vi "Facade 1.vi"(0 "Data In":T5, 2 "Display State In":T3, 3 "Container State":T4) -> (6 "Data Out":T5, 7 "Display State Out":T3, 8 "Action":T2)   [LabVIEW 2011, in "Calculator XControl.xctl"]
doc: "This VI defines the appearance and behavior of the Calculator XControl. The front panel of the Facade VI defines the appearance of the XControl. The block diagram of the Facade VI describes the behavior of the XControl, using an Event Structure to define responses to various events that can occur on the XControl."
uses:
  Calculator XControl.xctl
  Data 1.ctl
  <vilib>/_xctls/Container State.ctl
  State 1.ctl
  <vilib>/_xctls/Action.ctl
  Controls/Format.ctl
  <vilib>/event_ctls.llb/eventvkey.ctl
  <vilib>/_xctls/XControlSupport.lvlib
  <vilib>/gmath/NI_Gmath.lvlib
panel:
  out "Output":string
  in  "Backspace":bool
  in  "(":bool
  in  ")":bool
  in  "^":bool
  in  "E":bool
  in  "Tab Control":enum32{"Func", "Symbol"}(tab)
  in  "Cot":bool
  in  "Csc":bool
  in  "Sec":bool
  in  "e^":bool
  in  "tanh":bool
  in  "cosh":bool
  in  "sinh":bool
  in  "log":bool
  in  "ln":bool
  in  "Tan":bool
  in  "Cos":bool
  in  "Sin":bool
  in  "NA":bool
  in  "R":bool
  in  "c":bool
  in  "exp":bool
  in  "pi":bool
  in  "Answer":bool
  in  "Clear":bool
  in  "Precision":u8=6
  in  "Format":T1 items=["Decimal"=0, "Scientific"=1, "Hexadecimal"=5]
  in  "Equals":bool
  in  "Nine":bool
  in  "Eight":bool
  in  "Seven":bool
  in  "Six":bool
  in  "Five":bool
  in  "Four":bool
  in  "Decimal":bool
  in  "Three":bool
  in  "Two":bool
  in  "Zero":bool
  in  "One":bool
  in  "Divide":bool
  in  "Multiply":bool
  in  "Minus":bool
  in  "Plus":bool
  in  "Formula":string
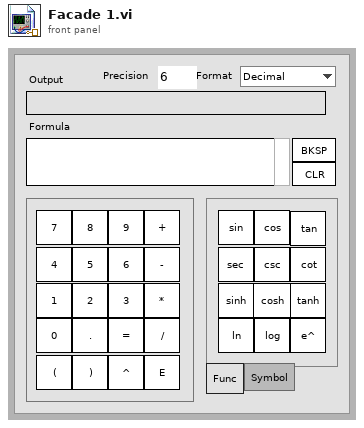
[diagram p1: front panel]
types:
  T1 = typedef "Calculator XControl.xctl/Format.ctl" = u16
  T2 = typedef "XControlSupport.lvlib/Action.ctl" = cluster{"Data Changed?":bool, "State Changed?":bool, "Action Name":string}
  T3 = typedef "Calculator XControl.xctl/State 1.ctl" = cluster{"Previous Formulas":string[]}
  T4 = typedef "XControlSupport.lvlib/Container State.ctl" = cluster{"Indicator?":bool, "Run Mode?":bool, " Refnum":refnum<vi>}
  T5 = typedef "Calculator XControl.xctl/Data 1.ctl" = dbl
  T6 = typedef "eventvkey.ctl" = enum16{"ASCII", "Enter", "Return", "Shift", "Ctrl", "Alt", "Cmd", "Opt", "Caps", "NumLock", "Clear", "Break", "Up", "Down", "Left", "Right", "Insert", "Delete", "Home", "End", "PageUp", "PageDown", "Escape", "Help", "Pause", "ScrollLock", "F1", "F2", "F3", "F4", "F5", "F6", "F7", "F8", "F9", "F10", "F11", "F12", "F13", "F14", "F15", "F16", "F17", "F18", "F19", "F20", "F21", "F22", "F23", "F24", "Play", "VolumeUp", "VolumeDown", "Mute", "Two Byte Char"}
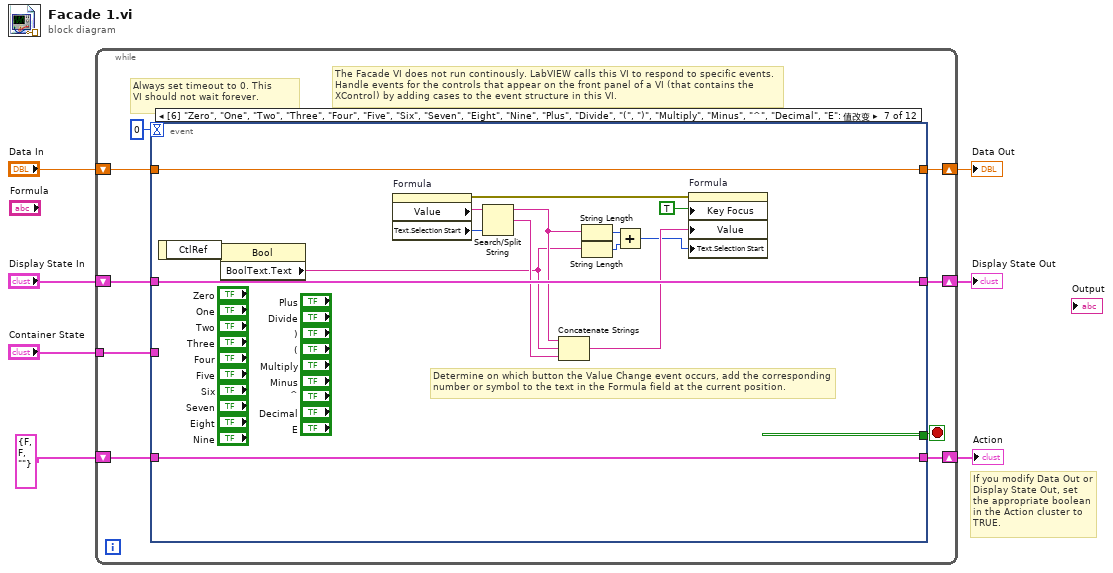
[diagram p0: block diagram]
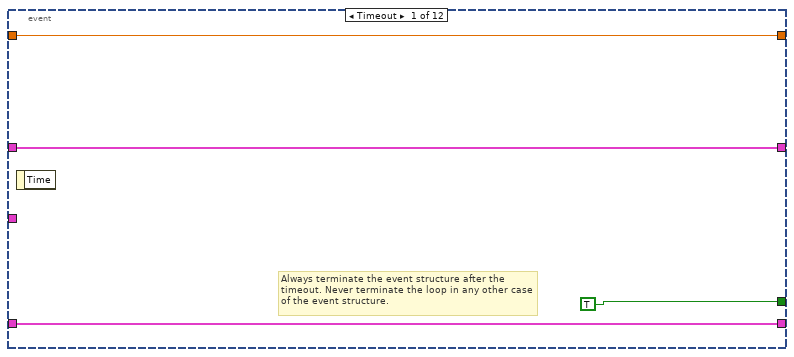
[diagram p2: hidden frame]
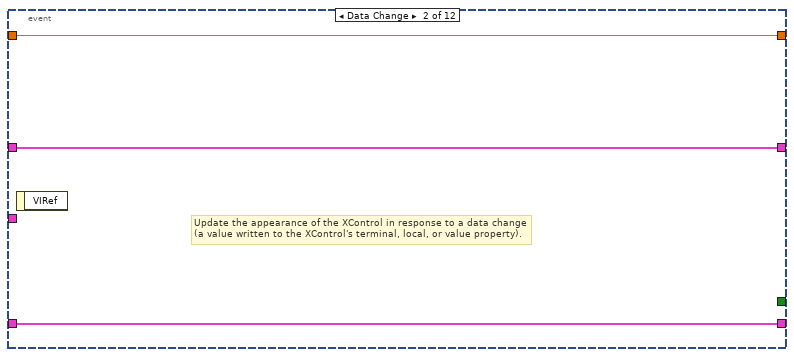
[diagram p3: hidden frame]
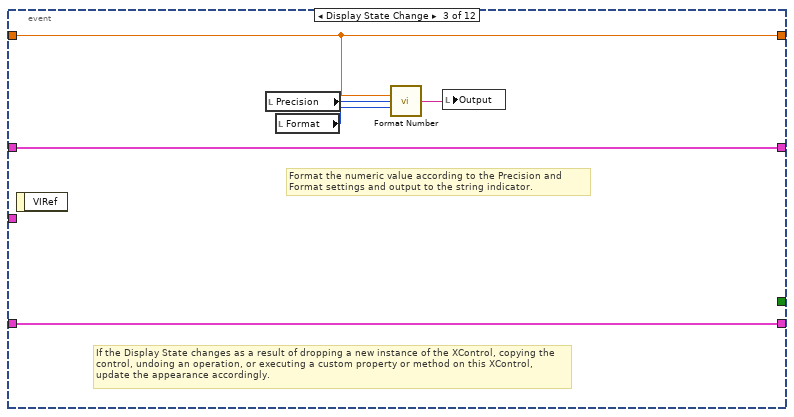
[diagram p4: hidden frame]
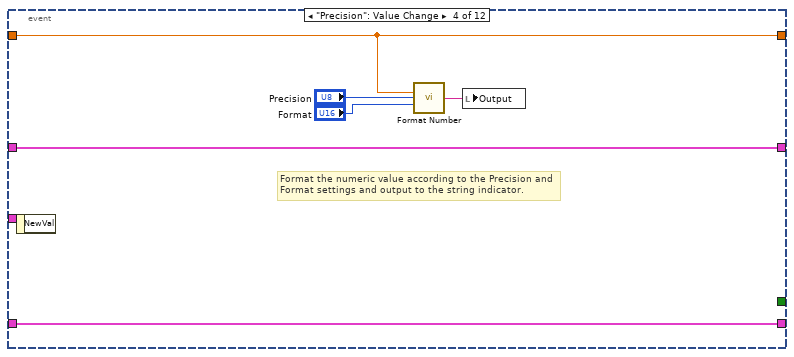
[diagram p5: hidden frame]
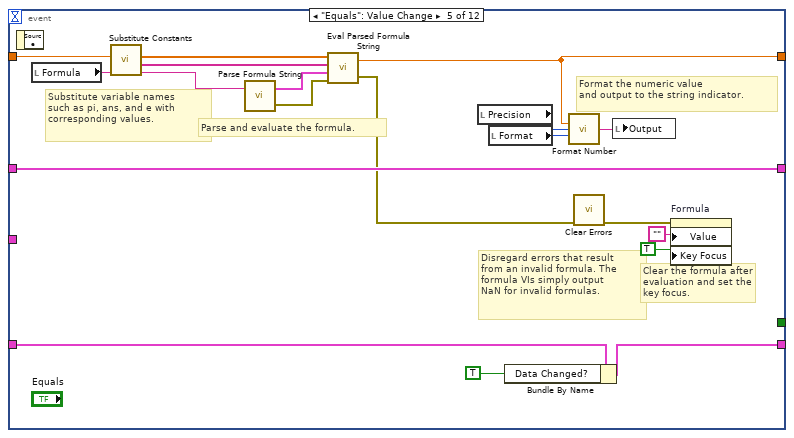
[diagram p6: hidden frame]
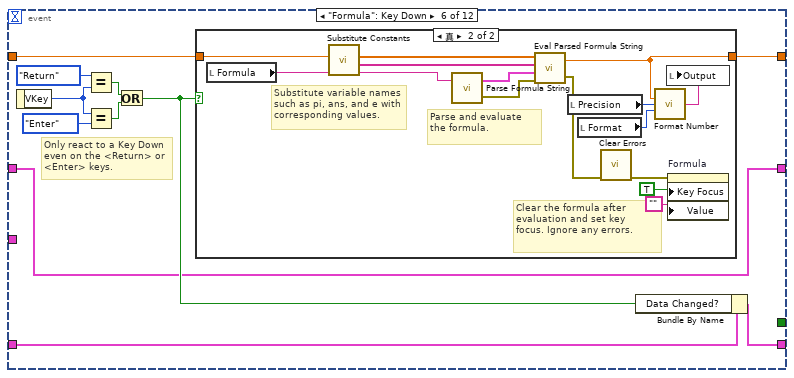
[diagram p7: hidden frame]
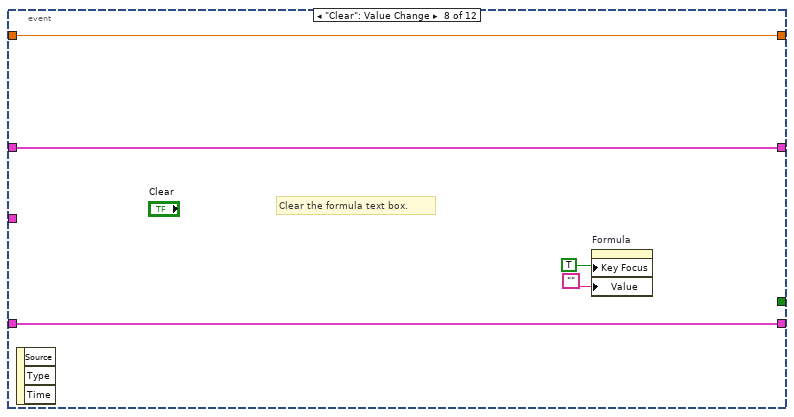
[diagram p9: hidden frame]
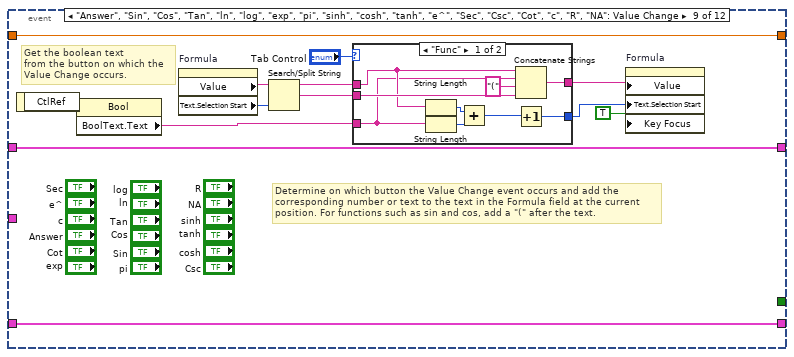
[diagram p10: hidden frame]
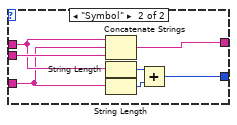
[diagram p11: hidden frame]
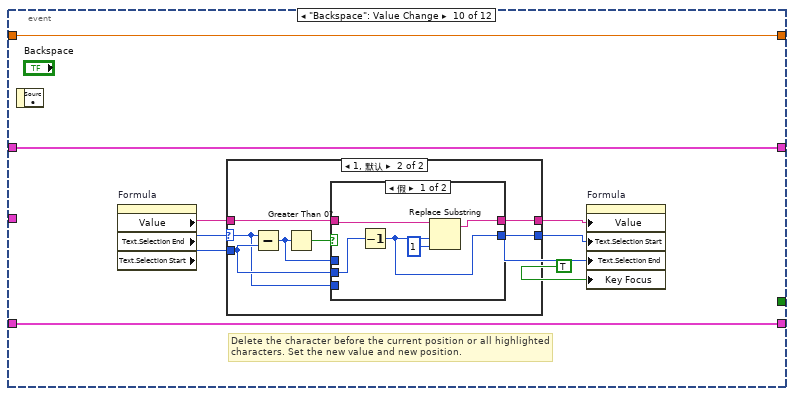
[diagram p12: hidden frame]
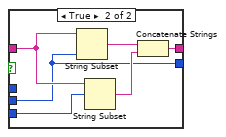
[diagram p14: hidden frame]
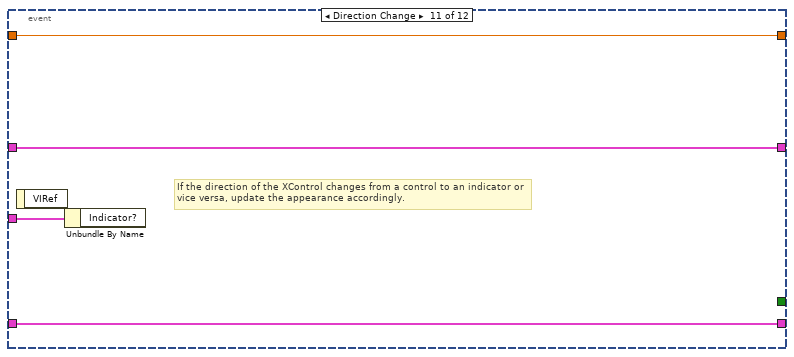
[diagram p15: hidden frame]
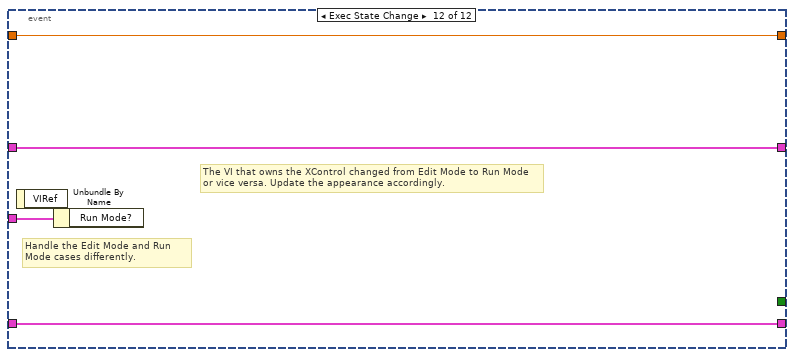
[diagram p16: hidden frame]
diagram:
  # "If you modify Data Out or Display State Out, set the appropriate boolean in the Action cluster to TRUE."
  n1 = while {
    shift-right: [w15] -> w4
    shift-left: "Display State In" -> [w16]
    tunnel: "Container State" -> [w12]
    shift-right: [w10] -> w7
    shift-left: "Data In" -> [w11]
    shift-right: [w8] -> w2
    shift-left: T2 {"Data Changed?"=FALSE, "State Changed?"=FALSE, "Action Name"=""} ("Action") -> [w9]
    stop <- w14 stop-if-true
    # "The Facade VI does not run continously. LabVIEW calls this VI to respond to specific events.  Handle events for the controls that appear on the front panel of a VI (that contains the XControl) by adding cases to the event structure in this VI."
    # "Always set timeout to 0. This\nVI should not wait forever."
    n2 = event shown="[6] \"Zero\", \"One\", \"Two\", \"Three\", \"Four\", \"Five\", \"Six\", \"Seven\", \"Eight\", \"Nine\", \"Plus\", \"Divide\", \"(\", \")\", \"Multiply\", \"Minus\", \"^\", \"Decimal\", \"E\": 值改变" {
      selector: _ -> [_ _ _ _ _ _ _ _ _ _ _ _]
      dyn-events: _ -> [_ _ _ _ _ _ _ _ _ _ _ _]
      timeout: 0 -> [_ _ _ _ _ _ _ _ _ _ _ _]
      tunnel: w16 -> [w18 w23 w28 w35 w42 w55 w95 w101 w113 w138 w162 w166]
      tunnel: [w18 w23 w28 w35 w42 w55 w95 w101 w113 w138 w162 w166] -> w15
      tunnel: [TRUE _ _ _ _ _ _ _ _ _ _ _] -> w14
      tunnel: w12 -> [_ _ _ _ _ _ _ _ _ _ w163 w167]
      tunnel: w11 -> [w17 w21 w27 w33 w47 w65 w94 w99 w114 w139 w161 w165]
      tunnel: [w17 w21 w27 w33 w37 w62 w94 w99 w114 w139 w161 w165] -> w10
      tunnel: [w19 w22 w29 w34 w51 w63 w96 w100 w112 w137 w160 w164] -> w8
      tunnel: w9 -> [w19 w22 w29 w34 w52 w64 w96 w100 w112 w137 w160 w164]
      event Timeout {
        # "Always terminate the event structure after the timeout. Never terminate the loop in any other case of the event structure."
        n3 = event-data() -> ()  [unwired: 1 in, 1 out]
      }
      event Data Change {
        # "Update the appearance of the XControl in response to a data change (a value written to the XControl's terminal, local, or value property)."
        n4 = event-data() -> ()  [unwired: 1 in, 1 out]
      }
      event Display State Change {
        # "Format the numeric value according to the Precision and Format settings and output to the string indicator."
        # "If the Display State changes as a result of dropping a new instance of the XControl, copying the control, undoing an operation, or executing a custom property or method on this XControl, update the appearance accordingly."
        n5 = event-data() -> ()  [unwired: 1 in, 1 out]
        n6 = local read "Precision"() -> (w25:u8)
        n7 = local read "Format"() -> (w26:T1)
        n8 = call "Format Number.vi"("Data"=w27, "precision (6)"=w25, "Format"=w26) -> ("Numeric String"=w24:string)  [unwired: 12 in]
        n9 = local write "Output"(w24) -> ()
      }
      event "Precision": Value Change {
        # "Format the numeric value according to the Precision and Format settings and output to the string indicator."
        n10 = event-data() -> ()  [unwired: 1 in, 1 out]
        n11 = call "Format Number.vi"("Data"=w33, "precision (6)"="Precision", "Format"="Format") -> ("Numeric String"=w30:string)  [unwired: 12 in]
        n12 = local write "Output"(w30) -> ()
      }
      event "Equals": Value Change {
        # "Format the numeric value\nand output to the string indicator."
        # "Disregard errors that result\nfrom an invalid formula. The\nformula VIs simply output\nNaN for invalid formulas."
        # "Clear the formula after\nevaluation and set the key focus."
        # "Parse and evaluate the formula."
        # "Substitute variable names\nsuch as pi, ans, and e with\ncorresponding values."
        n13 = event-data() -> ()  [unwired: 1 in, 1 out]
        n14 = local read "Formula"() -> (w44:string)
        n15 = call "Substitute Constants.vi"("Formula In"=w44, "Data In"=w47) -> ("Formula Out"=w43:string, "Variables Out"=w45:string[], "Values Out"=w46:dbl[])  [unwired: 7 in]
        n16 = call <vilib>:"Parse Formula String.vi"("formula"=w43) -> ("error out"=w54:errorcluster, "Parsed Formula"=w53:cluster{"Table":i32[][], "Y Values":dbl[]})  [unwired: 1 in]
        n17 = call <vilib>:"Eval Parsed Formula String.vi"("error in (no error)"=w54, "Parsed Formula"=w53, "Variables"=w45, "X Values"=w46) -> ("error out"=w41:errorcluster, "y value"=w37:dbl)
        n18 = local read "Precision"() -> (w38:u8)
        n19 = local read "Format"() -> (w39:T1)
        n20 = Bundle By Name(cluster=w52, "Data Changed?"=TRUE) -> (w51:T2)
        n21 = call "Format Number.vi"("Data"=w37, "precision (6)"=w38, "Format"=w39) -> ("Numeric String"=w36:string)  [unwired: 12 in]
        n22 = call <vilib>:"Clear Errors.vi"("error in (no error)"=w41) -> ("error out"=w40:errorcluster)  [unwired: 6 in]
        n23 = local write "Output"(w36) -> ()
        n24 = property on="Formula" class="Str"(error in=w40, "Value"="", "Key Focus"=TRUE) -> ()  [unwired: 1 in, 2 out]
      }
      event "Formula": Key Down {
        # "Only react to a Key Down even on the <Return> or <Enter> keys."
        n25 = event-data() -> ("VKey"=w60:T6)  [unwired: 1 in]
        n26 = Equal?(x=eventvkey."Return" ("y"), y=w60) -> (x = y?=w58:bool)
        n27 = Equal?(x=w60, y=eventvkey."Enter") -> (x = y?=w57:bool)
        n28 = Or(x=w58, y=w57) -> (x .or. y?=w56:bool)
        n29 = case shown="真" w56 {
          tunnel: w65 -> [w66 w77]
          tunnel: [w66 w70] -> w62
          frame False {
          }
          frame True {
            # "Clear the formula after\nevaluation and set key\nfocus. Ignore any errors."
            # "Substitute variable names\nsuch as pi, ans, and e with corresponding values."
            # "Parse and evaluate\nthe formula."
            n30 = local read "Formula"() -> (w74:string)
            n31 = call "Substitute Constants.vi"("Formula In"=w74, "Data In"=w77) -> ("Formula Out"=w73:string, "Variables Out"=w75:string[], "Values Out"=w76:dbl[])  [unwired: 7 in]
            n32 = call <vilib>:"Parse Formula String.vi"("formula"=w73) -> ("error out"=w81:errorcluster, "Parsed Formula"=w80:cluster{"Table":i32[][], "Y Values":dbl[]})  [unwired: 1 in]
            n33 = call <vilib>:"Eval Parsed Formula String.vi"("error in (no error)"=w81, "Parsed Formula"=w80, "Variables"=w75, "X Values"=w76) -> ("error out"=w72:errorcluster, "y value"=w70:dbl)
            n34 = local read "Precision"() -> (w69:u8)
            n35 = local read "Format"() -> (w68:T1)
            n36 = call <vilib>:"Clear Errors.vi"("error in (no error)"=w72) -> ("error out"=w71:errorcluster)  [unwired: 6 in]
            n37 = call "Format Number.vi"("Data"=w70, "precision (6)"=w69, "Format"=w68) -> ("Numeric String"=w67:string)  [unwired: 12 in]
            n38 = local write "Output"(w67) -> ()
            n39 = property on="Formula" class="Str"(error in=w71, "Key Focus"=TRUE, "Value"="") -> ()  [unwired: 1 in, 2 out]
          }
        }
        n40 = Bundle By Name(cluster=w64, "Data Changed?"=w56) -> (w63:T2)
      }
      event "Zero", "One", "Two", "Three", "Four", "Five", "Six", "Seven", "Eight", "Nine", "Plus", "Divide", "(", ")", "Multiply", "Minus", "^", "Decimal", "E": Value Change {
        # "Determine on which button the Value Change event occurs, add the corresponding number or symbol to the text in the Formula field at the current position."
        n41 = event-data() -> ("CtlRef"=w83:refnum<vi>)  [unwired: 1 in]
        n42 = property class="Bool"(reference=w83) -> ("BoolText.Text"=w82:string)  [unwired: 1 in, 2 out]
        n43 = property on="Formula" class="Str"() -> (error out=w90:errorcluster, "Value"=w93:string, "Text.Selection Start"=w92:u32)  [unwired: 2 in, 1 out]
        n44 = Search/Split String(string=w93, offset (0)=w92) -> (substring before match=w88:string, match + rest of string=w91:string)  [unwired: 1 in, 1 out]
        n45 = Concatenate Strings(w88, w82, w91) -> (w85:string)
        n46 = String Length(string=w88) -> (length=w87:i32)
        n47 = String Length(string=w82) -> (length=w86:i32)
        n48 = Add(x=w87, y=w86) -> (x+y=w84:i32)
        n49 = property on="Formula" class="Str"(error in=w90, "Key Focus"=TRUE, "Value"=w85, "Text.Selection Start"=w84) -> ()  [unwired: 1 in, 2 out]
      }
      event "Clear": Value Change {
        # "Clear the formula text box."
        n50 = event-data() -> ()  [unwired: 1 in, 3 out]
        n51 = property on="Formula" class="Str"("Key Focus"=TRUE, "Value"="") -> ()  [unwired: 2 in, 2 out]
      }
      event "Answer", "Sin", "Cos", "Tan", "ln", "log", "exp", "pi", "sinh", "cosh", "tanh", "e^", "Sec", "Csc", "Cot", "c", "R", "NA": Value Change {
        # "Get the boolean text\nfrom the button on which the Value Change occurs."
        # "Determine on which button the Value Change event occurs and add the corresponding number or text to the text in the Formula field at the current position. For functions such as sin and cos, add a \"(\" after the text."
        n52 = event-data() -> ("CtlRef"=w111:refnum<vi>)  [unwired: 1 in]
        n53 = property class="Bool"(reference=w111) -> ("BoolText.Text"=w103:string)  [unwired: 1 in, 2 out]
        n54 = property on="Formula" class="Str"() -> ("Value"=w110:string, "Text.Selection Start"=w109:u32)  [unwired: 2 in, 2 out]
        n55 = Search/Split String(string=w110, offset (0)=w109) -> (substring before match=w108:string, match + rest of string=w107:string)  [unwired: 1 in, 1 out]
        n56 = case shown="\"Func\"" "Tab Control" {
          tunnel: [w122 w130] -> w105
          tunnel: w108 -> [w120 w126]
          tunnel: w107 -> [w121 w129]
          tunnel: [w116 w125] -> w104
          tunnel: w103 -> [w115 w124]
          frame "Func" {
            n57 = String Length(string=w120) -> (length=w118:i32)
            n58 = String Length(string=w115) -> (length=w119:i32)
            n59 = Add(x=w118, y=w119) -> (x+y=w117:i32)
            n60 = Concatenate Strings(w120, w115, "(" ("string"), w121) -> (w122:string)
            n61 = Increment(x=w117) -> (x+1=w116:i32)
          }
          frame "Symbol" {
            n62 = Concatenate Strings(w126, w124, w129) -> (w130:string)
            n63 = String Length(string=w126) -> (length=w127:i32)
            n64 = String Length(string=w124) -> (length=w128:i32)
            n65 = Add(x=w127, y=w128) -> (x+y=w125:i32)
          }
        }
        n66 = property on="Formula" class="Str"("Value"=w105, "Text.Selection Start"=w104, "Key Focus"=TRUE) -> ()  [unwired: 2 in, 2 out]
      }
      event "Backspace": Value Change {
        # "Delete the character before the current position or all highlighted characters. Set the new value and new position."
        n67 = event-data() -> ()  [unwired: 1 in, 1 out]
        n68 = property on="Formula" class="Str"() -> ("Value"=w135:string, "Text.Selection End"=w131:u32, "Text.Selection Start"=w136:u32)  [unwired: 2 in, 2 out]
        n69 = case shown="1, 默认" w131 {
          selector: w131 -> [w140 w142]
          tunnel: w136 -> [_ w147]
          tunnel: w135 -> [w141 w146]
          tunnel: [w141 w144] -> w133
          tunnel: [w140 w143] -> w132
          frame 0 {
          }
          frame 1, Default {
            n70 = Subtract(x=w142, y=w147) -> (x-y=w145:u32)
            n71 = Greater Than 0?(x=w145) -> (x > 0?=w148:bool)
            n72 = case shown="假" w148 {
              tunnel: w147 -> [w150 w154]
              tunnel: w142 -> [_ w158]
              tunnel: w146 -> [w153 w159]
              tunnel: w145 -> [_ _]
              tunnel: [w151 w155] -> w144
              tunnel: [w149 w154] -> w143
              frame False {
                n73 = Decrement(x=w150) -> (x-1=w149:u32)
                n74 = Replace Substring(2:1 ("length (len. of substring)"), 3:w149, 5:w153) -> (1:w151:string)  [unwired: 1 in, 1 out]
              }
              frame True {
                n75 = String Subset(string=w159, length (rest)=w154) -> (substring=w157:string)  [unwired: 1 in]
                n76 = String Subset(string=w159, offset (0)=w158) -> (substring=w156:string)  [unwired: 1 in]
                n77 = Concatenate Strings(w157, w156) -> (w155:string)
              }
            }
          }
        }
        n78 = property on="Formula" class="Str"("Value"=w133, "Text.Selection Start"=w132, "Text.Selection End"=w132, "Key Focus"=TRUE) -> ()  [unwired: 2 in, 2 out]
      }
      event Direction Change {
        # "If the direction of the XControl changes from a control to an indicator or vice versa, update the appearance accordingly."
        n79 = event-data() -> ()  [unwired: 1 in, 1 out]
        n80 = Unbundle By Name(w163) -> ()  [unwired: 1 out]
      }
      event Exec State Change {
        # "The VI that owns the XControl changed from Edit Mode to Run Mode or vice versa. Update the appearance accordingly."
        # "Handle the Edit Mode and Run Mode cases differently."
        n81 = event-data() -> ()  [unwired: 1 in, 1 out]
        n82 = Unbundle By Name(w167) -> ()  [unwired: 1 out]
      }
    }
  }
  "Display State Out" <- w4
  "Data Out" <- w7
  "Action" <- w2
